vi "Set Temperature.vi"(8 "error in (no error)":errorcluster, 11 "CCDCamera in":refnum<class "iKon-L.lvclass">) -> (0 "error out":errorcluster, 3 "CCDCamera out":refnum<class "iKon-L.lvclass">)   [LabVIEW 2018, in "iKon-L.lvclass"]
doc: "Set the CCD temperature"
uses:
  iKon-L.lvclass
  C:/Users/Denis/Desktop/S4ACS/S4ACS/Sim_CCD/Sim_CCD.lvclass
  Sim_CCD/Sim_CCD.lvclass
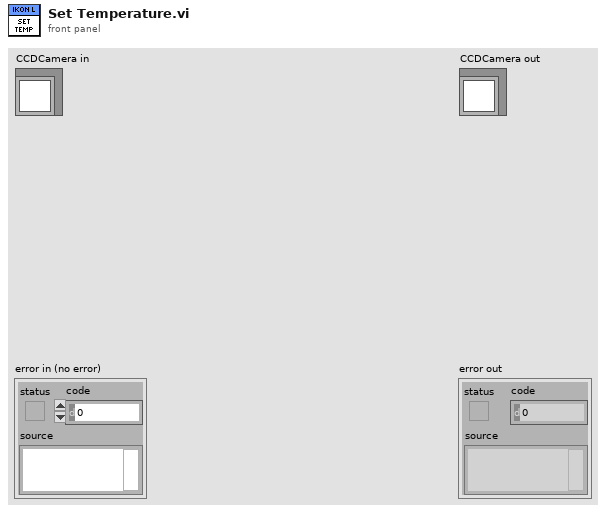
[diagram p1: front panel]
types:
  T1 = cluster{"EXPTIME":dbl, "#FRAMES":u32, "COOLER_POWER_STATUS":u16, "TEMP":i32}
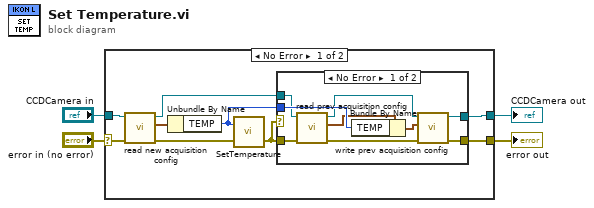
[diagram p0: block diagram]
diagram:
  n1 = case shown="No Error" "error in (no error)" {
    selector: "error in (no error)" -> [w9 w25]
    tunnel: "CCDCamera in" -> [w10 w26]
    tunnel: [w5 w26] -> w1
    tunnel: [w13 w25] -> w4
    frame No Error {
      n2 = call "read new acquisition config.vi"("error in (no error)"=w9, "Simulated_CCD_Camera in"=w10) -> ("error out"=w6:errorcluster, "new acquisition configuration"=w8:T1, "Simulated_CCD_Camera out"=w7:refnum<class "iKon-L.lvclass">)  [unwired: 7 in]
      n3 = Unbundle By Name(w8) -> ("TEMP"=w12:i32)
      n4 = call <userlib>:"SetTemperature.vi"("error in (no error)"=w6, "temperature"=w12) -> ("error out"=w11:errorcluster)  [unwired: 1 out]
      n5 = case shown="No Error" w11 {
        tunnel: [w17 w24] -> w13
        tunnel: w11 -> [w19 w24]
        tunnel: w12 -> [w22 _]
        tunnel: w7 -> [w20 w23]
        tunnel: [w16 w23] -> w5
        frame No Error {
          n6 = call "read prev acquisition config.vi"("error in (no error)"=w19, "Simulated_CCD_Camera in"=w20) -> ("error out"=w18:errorcluster, "prev acquisition configuration"=w15:T1, "Simulated_CCD_Camera out"=w21:refnum<class "iKon-L.lvclass">)  [unwired: 7 in]
          n7 = Bundle By Name(cluster=w15, "TEMP"=w22) -> (w14:T1)
          n8 = call "write prev acquisition config.vi"("error in (no error)"=w18, "prev acquisition configuration"=w14, "Simulated_CCD_Camera in"=w21) -> ("error out"=w17:errorcluster, "Simulated_CCD_Camera out"=w16:refnum<class "iKon-L.lvclass">)  [unwired: 7 in]
        }
        frame Error {
        }
      }
    }
    frame Error {
    }
  }
  "error out" <- w4
  "CCDCamera out" <- w1
